vi "Linear Profile.vi"(9 "dt":dbl, 10 "goal":dbl, 11 "v":dbl) -> (0 "X":dbl[](array[numeric]), 3 "V":dbl[](array[numeric]))   [LabVIEW 2020]
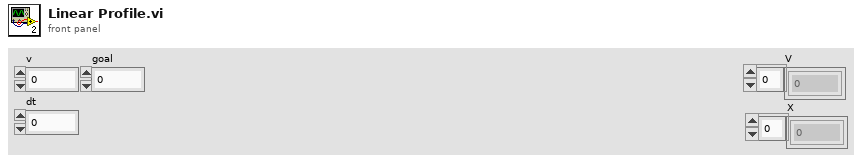
[diagram p1: front panel]
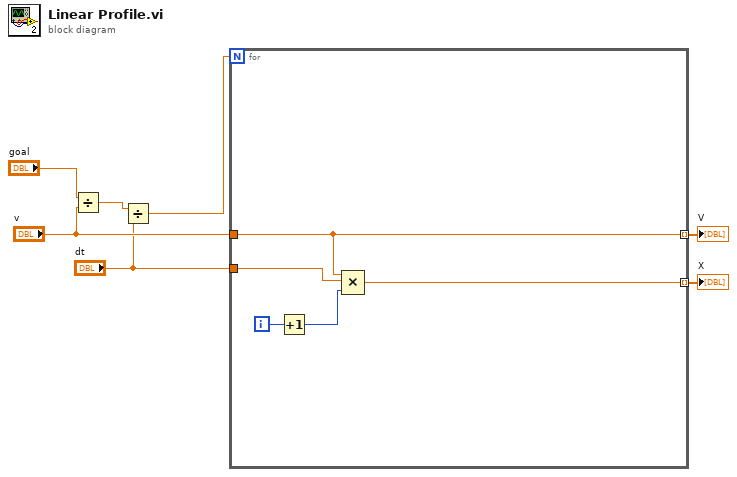
[diagram p0: block diagram]
diagram:
  n1 = Divide(x="goal", y="v") -> (x/y=w6:dbl)
  n2 = Divide(x=w6, y="dt") -> (x/y=w5:dbl)
  n3 = for {
    N: w5 -> [_]
    tunnel: [w11] -> w3 mode=indexing
    tunnel: "v" -> [w11]
    tunnel: "dt" -> [w10]
    tunnel: [w8] -> w1 mode=indexing
    i -> [w12]
    n4 = Increment(x=w12) -> (x+1=w9:i32)
    n5 = Compound Arithmetic op=MULTIPLY(w11, w10, w9) -> (w8:dbl)
  }
  "V" <- w3
  "X" <- w1
